vi "IO.vi"() -> ()   [LabVIEW 2020]
uses:
  Global_Variable/Global.vi
  Libraries/S7/S7.lvlib
panel:
  in  "选项卡控件":enum32{"DI", "DO", "伺服"}(tab)
  out "I 1":T1
  out "I 3":T2
  out "I 2":T3
  out "I 0":T4
  out "I 4":T5
  out "I 5":T6
  in  "Q5":T7
  in  "Q4":T8
  in  "Q3":T9
  in  "Q2":T10
  in  "Q1":T11
  in  "Q0":T12
  in  "输入轴旋转手动速度":sgl caption="手动速度" format="%#.3f"
  in  "输入轴旋转-正转":bool
  in  "输入轴旋转-反转":bool
  in  "输入轴旋转绝对位置":sgl caption="绝对位置" format="%#.3f"
  in  "输入轴旋转相对位置":sgl caption="相对位置" format="%#.3f"
  out "输入轴旋转当前位置":sgl caption="当前位置" format="%#.3f"
  in  "输入轴旋转-绝对定位":bool
  in  "输入轴旋转-相对定位":bool
  in  "输入轴移载手动速度":sgl caption="手动速度" format="%#.3f"
  in  "输入轴移载-正转":bool
  in  "输入轴移载-反转":bool
  in  "输入轴移载绝对位置":sgl caption="绝对位置" format="%#.3f"
  in  "输入轴移载相对位置":sgl caption="相对位置" format="%#.3f"
  out "输入轴移载当前位置":sgl caption="当前位置" format="%#.3f"
  in  "输入轴移载-绝对定位":bool
  in  "输入轴移载-相对定位":bool
  out "输出轴旋转当前位置":sgl caption="当前位置" format="%#.3f"
  in  "输出轴旋转-反转":bool
  in  "输出轴旋转-正转":bool
  in  "输出轴旋转手动速度":sgl caption="手动速度" format="%#.3f"
  in  "工装移载手动速度":sgl caption="手动速度" format="%#.3f"
  in  "工装移载-正转":bool
  in  "工装移载-反转":bool
  in  "工装移载绝对位置":sgl caption="绝对位置" format="%#.3f"
  in  "工装移载相对位置":sgl caption="相对位置" format="%#.3f"
  out "工装移载当前位置":sgl caption="当前位置" format="%#.3f"
  in  "工装移载-绝对定位":bool
  in  "工装移载-相对定位":bool
  out "输入轴旋转状态":bool
  out "输入轴移载状态":bool
  out "工装移载状态":bool
  out "输出轴旋转状态":bool
  out "输入扭矩":sgl format="%#.3f"
  out "输出扭矩(小)":sgl format="%#.3f"
  out "输出扭矩(大)":sgl format="%#.3f"
  out "吸收电流":sgl format="%#.3f"
  # "手动操作"
  # "输入轴旋转伺服"
  # "输出轴旋转伺服"
  # "输入轴移载伺服"
  # "工装移载伺服"
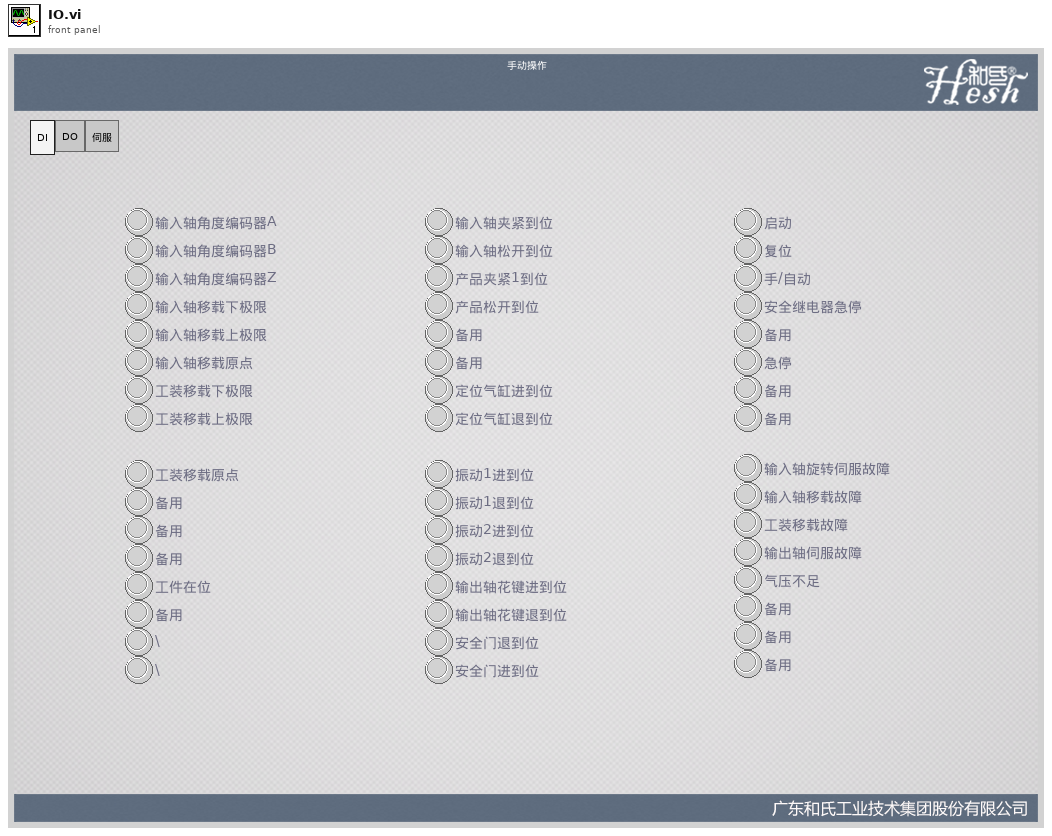
[diagram p1: front panel]
types:
  T1 = cluster{"工装移载原点":bool, "备用":bool, "备用":bool, "备用":bool, "工件在位":bool, "备用":bool, "\\":bool, "\\ ":bool}
  T2 = cluster{"振动1进到位":bool, "振动1退到位":bool, "振动2进到位":bool, "振动2退到位":bool, "输出轴花键进到位":bool, "输出轴花键退到位":bool, "安全门退到位":bool, "安全门进到位":bool}
  T3 = cluster{"输入轴夹紧到位":bool, "输入轴松开到位":bool, "产品夹紧1到位":bool, "产品松开到位":bool, "备用":bool, "备用":bool, "定位气缸进到位":bool, "定位气缸退到位":bool}
  T4 = cluster{"输入轴角度编码器A":bool, "输入轴角度编码器B":bool, "输入轴角度编码器Z":bool, "输入轴移载下极限":bool, "输入轴移载上极限":bool, "输入轴移载原点":bool, "工装移载下极限":bool, "工装移载上极限":bool}
  T5 = cluster{"启动":bool, "复位":bool, "手/自动":bool, "安全继电器急停":bool, "备用":bool, "急停":bool, "备用":bool, "备用":bool}
  T6 = cluster{"输入轴旋转伺服故障":bool, "输入轴移载故障":bool, "工装移载故障":bool, "输出轴伺服故障":bool, "气压不足":bool, "备用":bool, "备用":bool, "备用":bool}
  T7 = cluster{"备用":bool, "备用":bool, "备用":bool, "备用":bool, "备用":bool, "备用":bool, "备用":bool, "备用":bool}
  T8 = cluster{"三色灯-红":bool, "三色灯-黄":bool, "三色灯-绿":bool, "三色灯-蜂鸣器":bool, "不合格指示":bool, "合格指示":bool, "总气阀":bool, "备用":bool}
  T9 = cluster{"振动1进":bool, "振动1退":bool, "振动2进":bool, "振动2退":bool, "安全门退":bool, "安全门进":bool, "产品定位进":bool, "产品定位退":bool}
  T10 = cluster{"输入轴夹紧":bool, "输入轴松开":bool, "产品松开":bool, "产品夹紧":bool, "支架松开":bool, "支架夹紧":bool, "输出轴花键进":bool, "输出轴花键退":bool}
  T11 = cluster{"电机正转":bool, "电机反转":bool, "/":bool, "/":bool, "/":bool, "/":bool, "/":bool, "/":bool}
  T12 = cluster{"输入轴驱动Plus+":bool, "输入轴驱动Plus-":bool, "备用":bool, "点火信号":bool, "模拟转速":bool, "备用":bool, "模拟车速":bool, "备用":bool}
  T13 = cluster{bool, bool, bool, bool, bool, bool, bool, bool}
  T14 = typedef "S7.lvlib/Read_Data (Reply Payload)--cluster.ctl" = cluster{"读取成功":bool, "数据":u32[], "Read_Data_error":errorcluster}
  T15 = cluster{"Boolean array[0]":bool, "Boolean array[1]":bool, "Boolean array[2]":bool, "Boolean array[3]":bool, "Boolean array[4]":bool, "Boolean array[5]":bool, "Boolean array[6]":bool, "Boolean array[7]":bool}
  T16 = cluster{"输入旋转位移":sgl, "输入移载位移":sgl, "工装移载位移":sgl, "输入编码位移":sgl, "输入扭矩":sgl, "输出扭矩(小)":sgl, "输出扭矩(大)":sgl, "吸收电流":sgl}
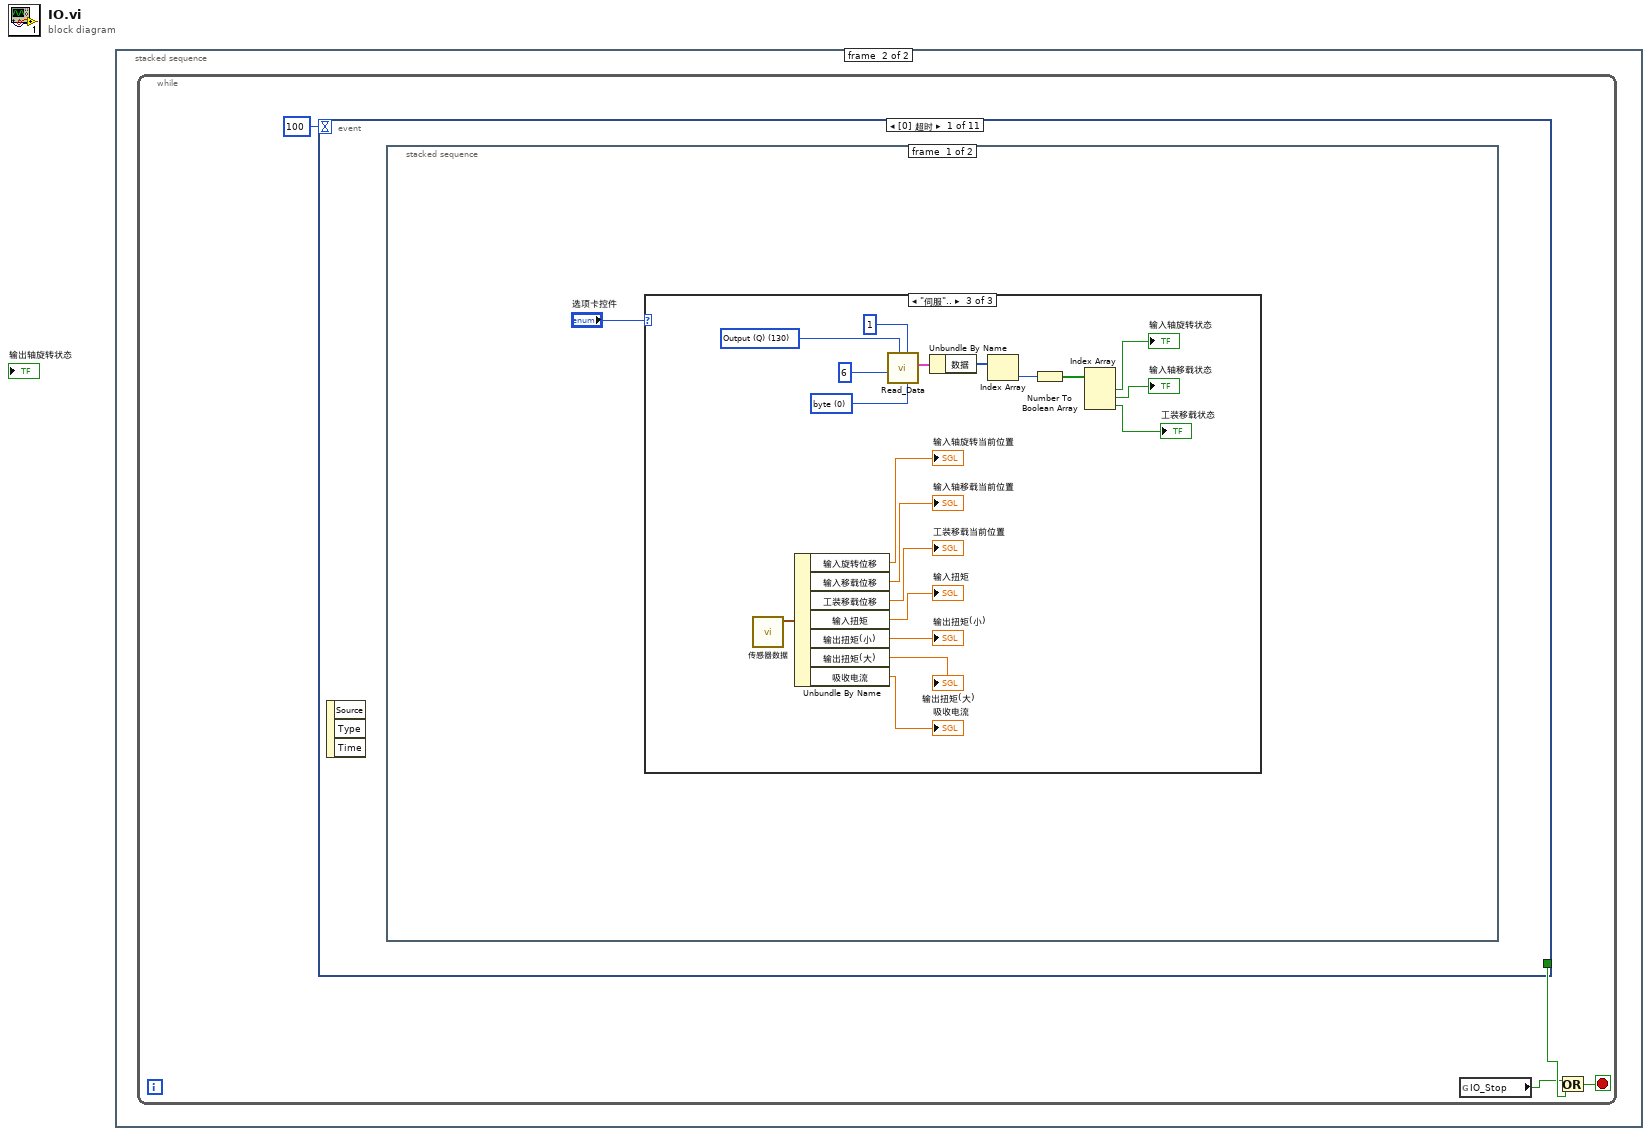
[diagram p0: block diagram]
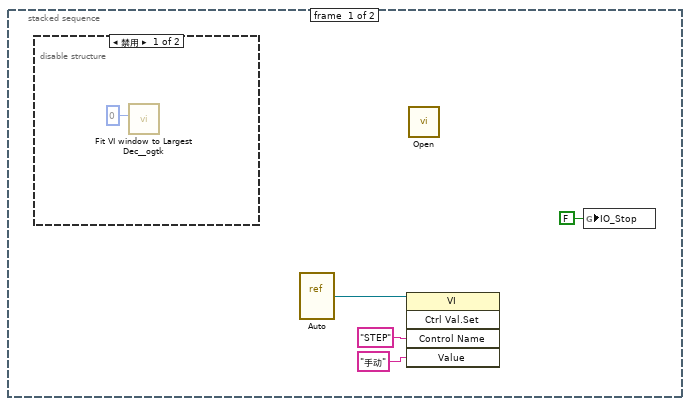
[diagram p2: hidden frame]
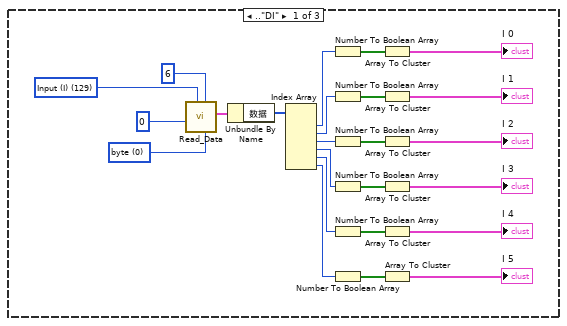
[diagram p4: hidden frame]
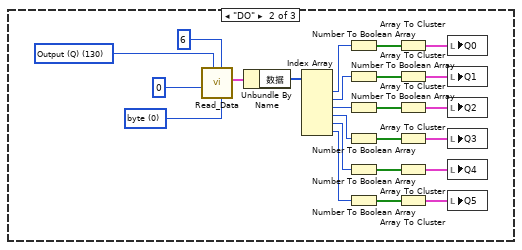
[diagram p5: hidden frame]
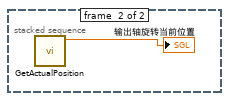
[diagram p6: hidden frame]
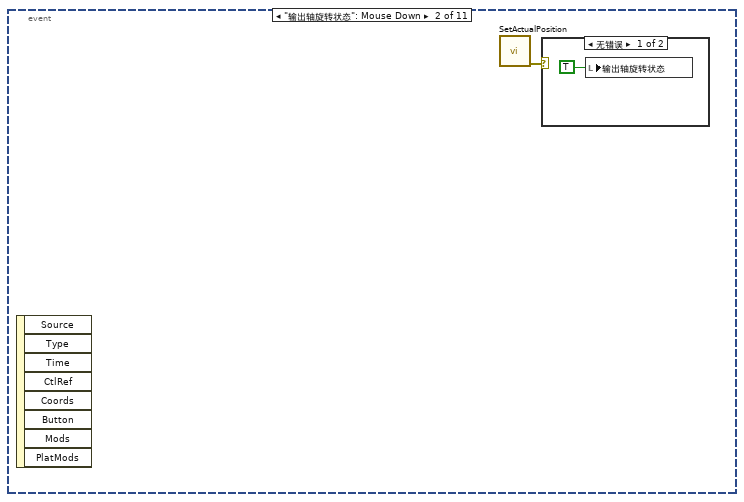
[diagram p7: hidden frame]
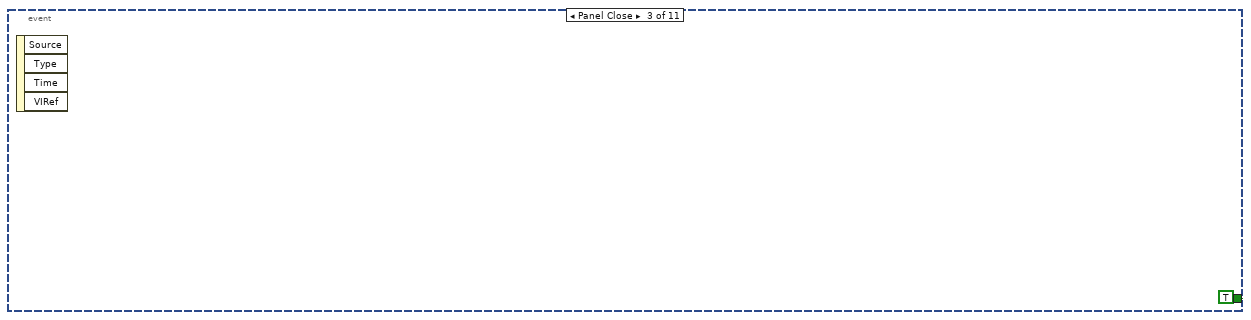
[diagram p9: hidden frame]
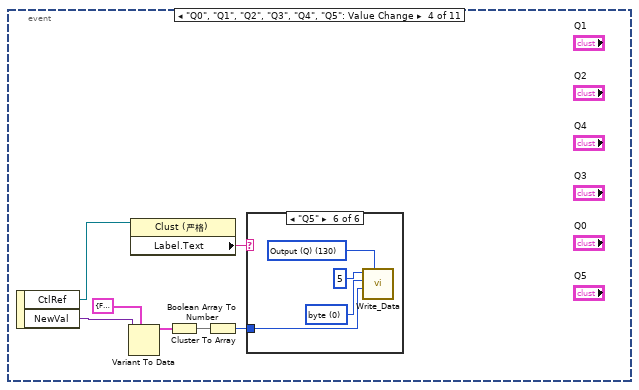
[diagram p10: hidden frame]
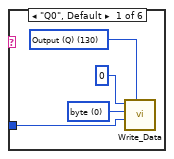
[diagram p11: hidden frame]
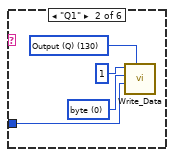
[diagram p12: hidden frame]
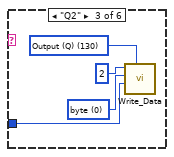
[diagram p13: hidden frame]
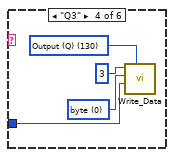
[diagram p14: hidden frame]
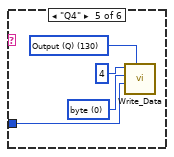
[diagram p15: hidden frame]
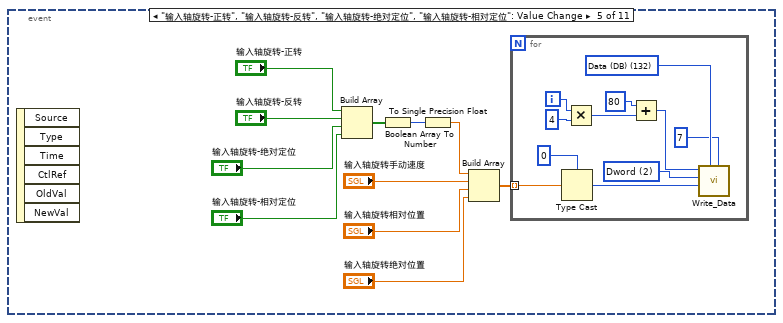
[diagram p16: hidden frame]
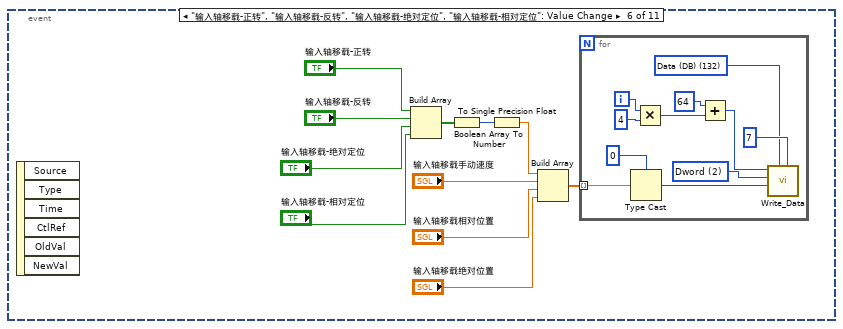
[diagram p17: hidden frame]
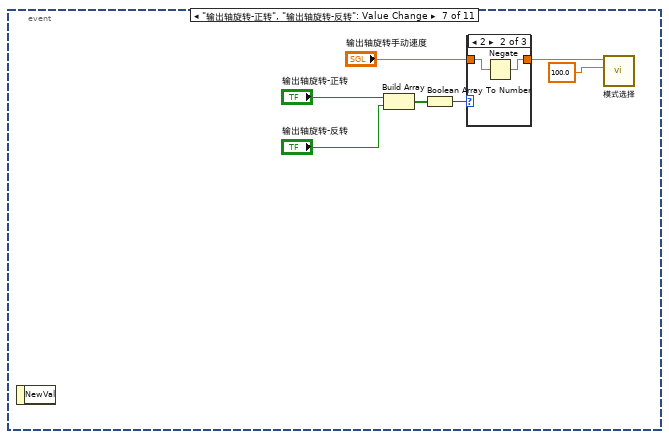
[diagram p18: hidden frame]
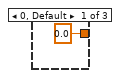
[diagram p19: hidden frame]
diagram:
  n1 = stacked-sequence {
    frame #0 {
      n2 = disable-structure shown="禁用" {
        frame Disabled {
          n3 = call <userlib>:"Fit VI window to Largest Dec__ogtk.vi"("border spacing (2 px)"=0) -> ()  [unwired: 5 in, 2 out]
        }
        frame Enabled {
        }
      }
      n4 = vi-ref "Auto.vi"() -> (w3:refnum<vi>)
      n5 = invoke class="VI" method="Ctrl Val.Set"(reference=w3, "Control Name"="STEP" ("控件名"), "Value"="手动" ("控件名")) -> ()  [unwired: 2 in, 5 out]
      n6 = call "Open.vi"() -> ()  [unwired: 11 in, 1 out]
      n7 = global write "Global.vi" "IO_Stop"(FALSE ("IO_Stop")) -> ()
    }
    frame #1 {
      n8 = while {
        stop <- w6 stop-if-true
        n9 = event shown="[0] 超时" {
          selector: _ -> [_ _ _ _ _ _ _ _ _ _ _]
          dyn-events: _ -> [_ _ _ _ _ _ _ _ _ _ _]
          timeout: 100 -> [_ _ _ _ _ _ _ _ _ _ _]
          tunnel: [_ _ TRUE _ _ _ _ _ _ _ _] -> w8
          event Timeout {
            n10 = event-data() -> ()  [unwired: 1 in, 3 out]
            n11 = stacked-sequence {
              frame #0 {
                n12 = case shown="\"伺服\".." "选项卡控件" {
                  frame .."DI" {
                    w14 = u16 0 items=["byte", "word", "Dword"] ("数据类型")
                    w12 = u8 129 items=["I/O (P)"=128, "Input (I)"=129, "Output (Q)"=130, "Bit Memory (M)"=131, "Data (DB)"=132, "Instance Data (DI)"=133, "Local Data (L)"=134, "Predecessor Local Data (VL)"=135] ("寄存器类型")
                    n13 = call "Read_Data.vi"("数据类型"=w14, "读取长度"=u16 6, "寄存器类型"=w12, "起始地址"=u32 0) -> ("Reply Payload"=w16:T14)  [unwired: 5 in, 2 out]
                    n14 = Unbundle By Name(w16) -> ("数据"=w15:u32[])
                    n15 = Index Array(array=w15) -> (element #1=w28:u32, element #2=w30:u32, element #3=w29:u32, element #4=w25:u32, element #5=w24:u32, element #6=w23:u32)  [unwired: 6 in]
                    n16 = Number To Boolean Array(number=w28) -> (Boolean array=w27:bool[])
                    n17 = Number To Boolean Array(number=w30) -> (Boolean array=w26:bool[])
                    n18 = Number To Boolean Array(number=w29) -> (Boolean array=w22:bool[])
                    n19 = Number To Boolean Array(number=w25) -> (Boolean array=w20:bool[])
                    n20 = Number To Boolean Array(number=w24) -> (Boolean array=w18:bool[])
                    n21 = Number To Boolean Array(number=w23) -> (Boolean array=w17:bool[])
                    n22 = Array To Cluster(array=w27) -> (cluster=→"I 0":T15)
                    n23 = Array To Cluster(array=w26) -> (cluster=→"I 1":T15)
                    n24 = Array To Cluster(array=w22) -> (cluster=→"I 2":T15)
                    n25 = Array To Cluster(array=w20) -> (cluster=→"I 3":T15)
                    n26 = Array To Cluster(array=w18) -> (cluster=→"I 4":T15)
                    n27 = Array To Cluster(array=w17) -> (cluster=→"I 5":T15)
                  }
                  frame "DO" {
                    w38 = u16 0 items=["byte", "word", "Dword"] ("数据类型")
                    w36 = u8 130 items=["I/O (P)"=128, "Input (I)"=129, "Output (Q)"=130, "Bit Memory (M)"=131, "Data (DB)"=132, "Instance Data (DI)"=133, "Local Data (L)"=134, "Predecessor Local Data (VL)"=135] ("寄存器类型")
                    n28 = call "Read_Data.vi"("数据类型"=w38, "读取长度"=u16 6, "寄存器类型"=w36, "起始地址"=u32 0) -> ("Reply Payload"=w57:T14)  [unwired: 5 in, 2 out]
                    n29 = Unbundle By Name(w57) -> ("数据"=w58:u32[])
                    n30 = Index Array(array=w58) -> (element #1=w48:u32, element #2=w50:u32, element #3=w49:u32, element #4=w47:u32, element #5=w46:u32, element #6=w45:u32)  [unwired: 6 in]
                    n31 = Number To Boolean Array(number=w48) -> (Boolean array=w51:bool[])
                    n32 = Number To Boolean Array(number=w50) -> (Boolean array=w52:bool[])
                    n33 = Number To Boolean Array(number=w49) -> (Boolean array=w53:bool[])
                    n34 = Number To Boolean Array(number=w47) -> (Boolean array=w54:bool[])
                    n35 = Number To Boolean Array(number=w46) -> (Boolean array=w55:bool[])
                    n36 = Number To Boolean Array(number=w45) -> (Boolean array=w56:bool[])
                    n37 = Array To Cluster(array=w51) -> (cluster=w43:T15)
                    n38 = Array To Cluster(array=w52) -> (cluster=w44:T15)
                    n39 = Array To Cluster(array=w53) -> (cluster=w41:T15)
                    n40 = Array To Cluster(array=w54) -> (cluster=w42:T15)
                    n41 = Array To Cluster(array=w55) -> (cluster=w40:T15)
                    n42 = Array To Cluster(array=w56) -> (cluster=w39:T15)
                    n43 = local write "Q0"(w43) -> ()
                    n44 = local write "Q1"(w44) -> ()
                    n45 = local write "Q2"(w41) -> ()
                    n46 = local write "Q3"(w42) -> ()
                    n47 = local write "Q4"(w40) -> ()
                    n48 = local write "Q5"(w39) -> ()
                  }
                  frame "伺服".. {
                    w70 = u16 0 items=["byte", "word", "Dword"] ("数据类型")
                    w68 = u8 130 items=["I/O (P)"=128, "Input (I)"=129, "Output (Q)"=130, "Bit Memory (M)"=131, "Data (DB)"=132, "Instance Data (DI)"=133, "Local Data (L)"=134, "Predecessor Local Data (VL)"=135] ("寄存器类型")
                    n49 = call "传感器数据.vi"() -> ("传感器读数"=w62:T16)  [unwired: 11 in]
                    n50 = Unbundle By Name(w62) -> ("输入旋转位移"=→"输入轴旋转当前位置":sgl, "输入移载位移"=→"输入轴移载当前位置":sgl, "工装移载位移"=→"工装移载当前位置":sgl, "输入扭矩"=→"输入扭矩":sgl, "输出扭矩(小)"=→"输出扭矩(小)":sgl, "输出扭矩(大)"=→"输出扭矩(大)":sgl, "吸收电流"=→"吸收电流":sgl)
                    n51 = call "Read_Data.vi"("数据类型"=w70, "读取长度"=u16 1, "寄存器类型"=w68, "起始地址"=u32 6) -> ("Reply Payload"=w71:T14)  [unwired: 5 in, 2 out]
                    n52 = Unbundle By Name(w71) -> ("数据"=w72:u32[])
                    n53 = Index Array(array=w72) -> (element=w77:u32)  [unwired: 1 in]
                    n54 = Number To Boolean Array(number=w77) -> (Boolean array=w74:bool[])
                    n55 = Index Array(array=w74) -> (element #1=→"输入轴旋转状态":bool, element #2=→"输入轴移载状态":bool, element #3=→"工装移载状态":bool)  [unwired: 3 in]
                  }
                }
              }
              frame #1 {
                n56 = call "GetActualPosition.vi"() -> ("Axis_ActualPosition(°)"=→"输出轴旋转当前位置":dbl)  [unwired: 11 in]
              }
            }
          }
          event "输出轴旋转状态": Mouse Down {
            n57 = event-data() -> ()  [unwired: 1 in, 8 out]
            n58 = call "SetActualPosition.vi"() -> ("error out"=w79:errorcluster)  [unwired: 11 in]
            n59 = case shown="无错误" w79 {
              frame No Error {
                n60 = local write "输出轴旋转状态"(TRUE ("输出轴旋转状态")) -> ()
              }
              frame Error {
              }
            }
          }
          event Panel Close {
            n61 = event-data() -> ()  [unwired: 1 in, 4 out]
          }
          event "Q0", "Q1", "Q2", "Q3", "Q4", "Q5": Value Change {
            n62 = event-data() -> ("CtlRef"=w83:refnum<vi>, "NewVal"=w87:variant)  [unwired: 1 in]
            n63 = Variant To Data(type=T13 {FALSE, FALSE, FALSE, FALSE, FALSE, FALSE, FALSE, FALSE}, Variant=w87) -> (data=w86:T13)  [unwired: 1 in, 1 out]
            n64 = property class="Clust (严格)"(reference=w83) -> ("Label.Text"=w82:string)  [unwired: 1 in, 2 out]
            n65 = Cluster To Array(cluster=w86) -> (array=w85:bool[])
            n66 = Boolean Array To Number(Boolean array=w85) -> (number=w84:u32)
            n67 = case shown="\"Q5\"" w82 {
              tunnel: w84 -> [w92 w96 w100 w104 w108 w112]
              frame "Q0", Default {
                w90 = u16 0 items=["byte", "word", "Dword"] ("数据类型")
                w91 = u8 130 items=["I/O (P)"=128, "Input (I)"=129, "Output (Q)"=130, "Bit Memory (M)"=131, "Data (DB)"=132, "Instance Data (DI)"=133, "Local Data (L)"=134, "Predecessor Local Data (VL)"=135] ("寄存器类型")
                n68 = call "Write_Data.vi"("寄存器类型"=w91, "写入数据"=w92, "数据类型"=w90, "写入地址"=u32 0) -> ()  [unwired: 5 in, 3 out]
              }
              frame "Q1" {
                w94 = u16 0 items=["byte", "word", "Dword"] ("数据类型")
                w95 = u8 130 items=["I/O (P)"=128, "Input (I)"=129, "Output (Q)"=130, "Bit Memory (M)"=131, "Data (DB)"=132, "Instance Data (DI)"=133, "Local Data (L)"=134, "Predecessor Local Data (VL)"=135] ("寄存器类型")
                n69 = call "Write_Data.vi"("寄存器类型"=w95, "写入数据"=w96, "数据类型"=w94, "写入地址"=u32 1) -> ()  [unwired: 5 in, 3 out]
              }
              frame "Q2" {
                w98 = u16 0 items=["byte", "word", "Dword"] ("数据类型")
                w99 = u8 130 items=["I/O (P)"=128, "Input (I)"=129, "Output (Q)"=130, "Bit Memory (M)"=131, "Data (DB)"=132, "Instance Data (DI)"=133, "Local Data (L)"=134, "Predecessor Local Data (VL)"=135] ("寄存器类型")
                n70 = call "Write_Data.vi"("寄存器类型"=w99, "写入数据"=w100, "数据类型"=w98, "写入地址"=u32 2) -> ()  [unwired: 5 in, 3 out]
              }
              frame "Q3" {
                w102 = u16 0 items=["byte", "word", "Dword"] ("数据类型")
                w103 = u8 130 items=["I/O (P)"=128, "Input (I)"=129, "Output (Q)"=130, "Bit Memory (M)"=131, "Data (DB)"=132, "Instance Data (DI)"=133, "Local Data (L)"=134, "Predecessor Local Data (VL)"=135] ("寄存器类型")
                n71 = call "Write_Data.vi"("寄存器类型"=w103, "写入数据"=w104, "数据类型"=w102, "写入地址"=u32 3) -> ()  [unwired: 5 in, 3 out]
              }
              frame "Q4" {
                w106 = u16 0 items=["byte", "word", "Dword"] ("数据类型")
                w107 = u8 130 items=["I/O (P)"=128, "Input (I)"=129, "Output (Q)"=130, "Bit Memory (M)"=131, "Data (DB)"=132, "Instance Data (DI)"=133, "Local Data (L)"=134, "Predecessor Local Data (VL)"=135] ("寄存器类型")
                n72 = call "Write_Data.vi"("寄存器类型"=w107, "写入数据"=w108, "数据类型"=w106, "写入地址"=u32 4) -> ()  [unwired: 5 in, 3 out]
              }
              frame "Q5" {
                w110 = u16 0 items=["byte", "word", "Dword"] ("数据类型")
                w111 = u8 130 items=["I/O (P)"=128, "Input (I)"=129, "Output (Q)"=130, "Bit Memory (M)"=131, "Data (DB)"=132, "Instance Data (DI)"=133, "Local Data (L)"=134, "Predecessor Local Data (VL)"=135] ("寄存器类型")
                n73 = call "Write_Data.vi"("寄存器类型"=w111, "写入数据"=w112, "数据类型"=w110, "写入地址"=u32 5) -> ()  [unwired: 5 in, 3 out]
              }
            }
          }
          event "输入轴旋转-正转", "输入轴旋转-反转", "输入轴旋转-绝对定位", "输入轴旋转-相对定位": Value Change {
            n74 = event-data() -> ()  [unwired: 1 in, 6 out]
            n75 = Build Array("输入轴旋转-正转", "输入轴旋转-反转", "输入轴旋转-绝对定位", "输入轴旋转-相对定位") -> (w122:bool[])
            n76 = Boolean Array To Number(Boolean array=w122) -> (number=w121:u32)
            n77 = To Single Precision Float(number=w121) -> (single precision float=w123:sgl)
            n78 = Build Array(w123, "输入轴旋转手动速度", "输入轴旋转相对位置", "输入轴旋转绝对位置") -> (w120:sgl[])
            n79 = for {
              tunnel: w120 -> [w129] mode=indexing
              i -> [w126]
              w131 = u16 2 items=["byte", "word", "Dword"] ("数据类型")
              w134 = u8 132 items=["I/O (P)"=128, "Input (I)"=129, "Output (Q)"=130, "Bit Memory (M)"=131, "Data (DB)"=132, "Instance Data (DI)"=133, "Local Data (L)"=134, "Predecessor Local Data (VL)"=135] ("寄存器类型")
              n80 = Type Cast(type=u32 0, x=w129) -> (*(type *) &x=w128:u32)
              n81 = Multiply(x=w126, y=u32 4) -> (x*y=w125:u32)
              n82 = Add(x=u32 80 ("写入地址"), y=w125) -> (x+y=w124:u32)
              n83 = call "Write_Data.vi"("DB #"=u16 7, "寄存器类型"=w134, "写入数据"=w128, "数据类型"=w131, "写入地址"=w124) -> ()  [unwired: 4 in, 3 out]
            }
          }
          event "输入轴移载-正转", "输入轴移载-反转", "输入轴移载-绝对定位", "输入轴移载-相对定位": Value Change {
            n84 = event-data() -> ()  [unwired: 1 in, 6 out]
            n85 = Build Array("输入轴移载-正转", "输入轴移载-反转", "输入轴移载-绝对定位", "输入轴移载-相对定位") -> (w144:bool[])
            n86 = Boolean Array To Number(Boolean array=w144) -> (number=w143:u32)
            n87 = To Single Precision Float(number=w143) -> (single precision float=w145:sgl)
            n88 = Build Array(w145, "输入轴移载手动速度", "输入轴移载相对位置", "输入轴移载绝对位置") -> (w142:sgl[])
            n89 = for {
              tunnel: w142 -> [w154] mode=indexing
              i -> [w152]
              w147 = u16 2 items=["byte", "word", "Dword"] ("数据类型")
              w149 = u8 132 items=["I/O (P)"=128, "Input (I)"=129, "Output (Q)"=130, "Bit Memory (M)"=131, "Data (DB)"=132, "Instance Data (DI)"=133, "Local Data (L)"=134, "Predecessor Local Data (VL)"=135] ("寄存器类型")
              n90 = Type Cast(type=u32 0, x=w154) -> (*(type *) &x=w146:u32)
              n91 = Multiply(x=w152, y=u32 4) -> (x*y=w151:u32)
              n92 = Add(x=u32 64 ("写入地址"), y=w151) -> (x+y=w148:u32)
              n93 = call "Write_Data.vi"("DB #"=u16 7, "寄存器类型"=w149, "写入数据"=w146, "数据类型"=w147, "写入地址"=w148) -> ()  [unwired: 4 in, 3 out]
            }
          }
          event "输出轴旋转-正转", "输出轴旋转-反转": Value Change {
            n94 = event-data() -> ()  [unwired: 1 in, 1 out]
            n95 = Build Array("输出轴旋转-正转", "输出轴旋转-反转") -> (w158:bool[])
            n96 = Boolean Array To Number(Boolean array=w158) -> (number=w157:u32)
            n97 = case shown="2" w157 {
              tunnel: "输出轴旋转手动速度" -> [_ w166 w167]
              tunnel: [sgl 0.0 ("输出轴旋转手动速度") w165 w167] -> w161
              frame 0, Default {
              }
              frame 2 {
                n98 = Negate(x=w166) -> (-x=w165:sgl)
              }
              frame 1 {
              }
            }
            n99 = call-poly "模式选择.vi"("Max Torque"=100.0, "Velocity"=w161) -> ()  [unwired: 9 in, 1 out]
          }
          event "输入轴旋转状态": Mouse Down {
            w170 = u16 2 items=["byte", "word", "Dword"] ("数据类型")
            w172 = u8 132 items=["I/O (P)"=128, "Input (I)"=129, "Output (Q)"=130, "Bit Memory (M)"=131, "Data (DB)"=132, "Instance Data (DI)"=133, "Local Data (L)"=134, "Predecessor Local Data (VL)"=135] ("寄存器类型")
            n100 = event-data() -> ()  [unwired: 1 in, 1 out]
            n101 = Type Cast(type=u32 0, x=sgl 16.0) -> (*(type *) &x=w174:u32)
            n102 = call "Write_Data.vi"("DB #"=u16 7, "寄存器类型"=w172, "写入数据"=w174, "数据类型"=w170, "写入地址"=u32 80) -> ()  [unwired: 4 in, 3 out]
          }
          event "输入轴移载状态": Mouse Down {
            w175 = u16 2 items=["byte", "word", "Dword"] ("数据类型")
            w178 = u8 132 items=["I/O (P)"=128, "Input (I)"=129, "Output (Q)"=130, "Bit Memory (M)"=131, "Data (DB)"=132, "Instance Data (DI)"=133, "Local Data (L)"=134, "Predecessor Local Data (VL)"=135] ("寄存器类型")
            n103 = event-data() -> ()  [unwired: 1 in, 1 out]
            n104 = Type Cast(type=u32 0, x=sgl 16.0) -> (*(type *) &x=w181:u32)
            n105 = call "Write_Data.vi"("DB #"=u16 7, "寄存器类型"=w178, "写入数据"=w181, "数据类型"=w175, "写入地址"=u32 64) -> ()  [unwired: 4 in, 3 out]
          }
          event "工装移载状态": Mouse Down {
            w182 = u16 2 items=["byte", "word", "Dword"] ("数据类型")
            w185 = u8 132 items=["I/O (P)"=128, "Input (I)"=129, "Output (Q)"=130, "Bit Memory (M)"=131, "Data (DB)"=132, "Instance Data (DI)"=133, "Local Data (L)"=134, "Predecessor Local Data (VL)"=135] ("寄存器类型")
            n106 = event-data() -> ()  [unwired: 1 in, 1 out]
            n107 = Type Cast(type=u32 0, x=sgl 16.0) -> (*(type *) &x=w188:u32)
            n108 = call "Write_Data.vi"("DB #"=u16 7, "寄存器类型"=w185, "写入数据"=w188, "数据类型"=w182, "写入地址"=u32 104) -> ()  [unwired: 4 in, 3 out]
          }
          event "工装移载-正转", "工装移载-反转", "工装移载-绝对定位", "工装移载-相对定位": Value Change {
            n109 = event-data() -> ()  [unwired: 1 in, 6 out]
            n110 = Build Array("工装移载-正转", "工装移载-反转", "工装移载-绝对定位", "工装移载-相对定位") -> (w195:bool[])
            n111 = Boolean Array To Number(Boolean array=w195) -> (number=w194:u32)
            n112 = To Single Precision Float(number=w194) -> (single precision float=w193:sgl)
            n113 = Build Array(w193, "工装移载手动速度", "工装移载相对位置", "工装移载绝对位置") -> (w191:sgl[])
            n114 = for {
              tunnel: w191 -> [w205] mode=indexing
              i -> [w202]
              w207 = u16 2 items=["byte", "word", "Dword"] ("数据类型")
              w210 = u8 132 items=["I/O (P)"=128, "Input (I)"=129, "Output (Q)"=130, "Bit Memory (M)"=131, "Data (DB)"=132, "Instance Data (DI)"=133, "Local Data (L)"=134, "Predecessor Local Data (VL)"=135] ("寄存器类型")
              n115 = Type Cast(type=u32 0, x=w205) -> (*(type *) &x=w204:u32)
              n116 = Multiply(x=w202, y=u32 4) -> (x*y=w201:u32)
              n117 = Add(x=u32 104 ("写入地址"), y=w201) -> (x+y=w200:u32)
              n118 = call "Write_Data.vi"("DB #"=u16 7, "寄存器类型"=w210, "写入数据"=w204, "数据类型"=w207, "写入地址"=w200) -> ()  [unwired: 4 in, 3 out]
            }
          }
        }
        n119 = global read "Global.vi" "IO_Stop"() -> (w7:bool)
        n120 = Or(x=w7, y=w8) -> (x .or. y?=w6:bool)
      }
    }
  }
